vi "Add Injector Commands Section.vi"(8 "error in (no error)":errorcluster, 9 "Default Current Offset":dbl, 10 "Default Volt Offset":dbl, 11 "Injector Section ptr":T1=18446744073709551615 format="%.0x") -> (0 "error out":errorcluster, 3 "Parent Ref out":T1 format="%.0x")   [LabVIEW 2019, in "Fuel Injector Analysis Addon System Explorer.lvlib"]
uses:
  Fuel Injector Analysis Addon System Explorer.lvlib
  <vilib>/NI VeriStand/Custom Device API/Custom Device Item Ref.ctl
  <vilib>/NI VeriStand/Custom Device API/Custom Device Channel.ctl
  <vilib>/NI VeriStand/Custom Device API/Custom Device Channel Type.ctl
  Addon Shared/SubVIs/Constants.vi
  <vilib>/NI VeriStand/Custom Device API/Custom Device API.lvlib
  Addon Shared/Fuel Injector Analysis Addon Shared.lvlib
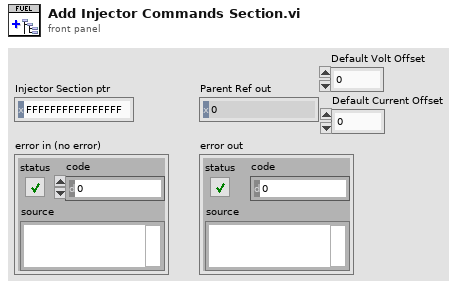
[diagram p1: front panel]
types:
  T1 = typedef "Custom Device API.lvlib/Custom Device Item Ref.ctl" = u64
  T2 = typedef "Custom Device API.lvlib/Custom Device Channel.ctl" = cluster{"Type":T3, "Units":string, "Default Value":dbl, "Faultable":bool, "Scalable":bool}
  T3 = typedef "Custom Device API.lvlib/Custom Device Channel Type.ctl" = enum16{"Input", "Output"}
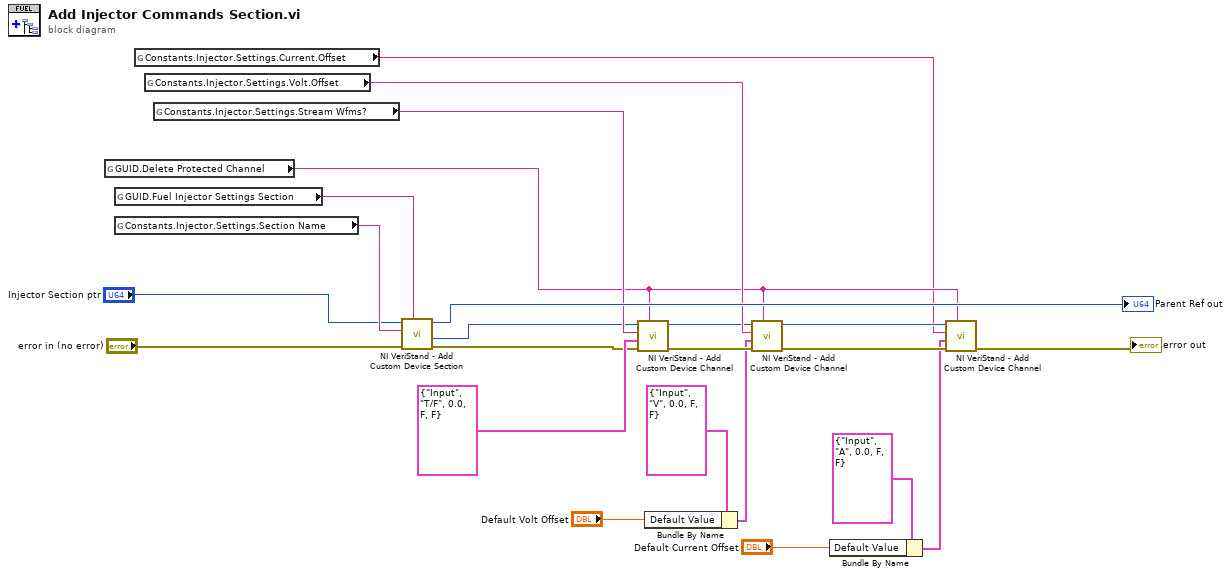
[diagram p0: block diagram]
diagram:
  n1 = global read "Constants.vi" "GUID.Delete Protected Channel"() -> (w8:string)
  n2 = global read "Constants.vi" "GUID.Fuel Injector Settings Section"() -> (w20:string)
  n3 = global read "Constants.vi" "Constants.Injector.Settings.Section Name"() -> (w19:string)
  n4 = global read "Constants.vi" "Constants.Injector.Settings.Current.Offset"() -> (w7:string)
  n5 = global read "Constants.vi" "Constants.Injector.Settings.Volt.Offset"() -> (w15:string)
  n6 = global read "Constants.vi" "Constants.Injector.Settings.Stream Wfms?"() -> (w21:string)
  n7 = call <vilib>:"NI VeriStand - Add Custom Device Section.vi"("GUID (Default Section)"=w20, "error in (no error)"="error in (no error)", "Section Name"=w19, "Parent Ref in"="Injector Section ptr") -> ("error out"=w13:errorcluster, "Section Ptr"=w12:T1, "Parent Ref out"=→"Parent Ref out":T1)  [unwired: 4 in, 1 out]
  n8 = call <vilib>:"NI VeriStand - Add Custom Device Channel.vi"("GUID (Default Channel)"=w8, "error in (no error)"=w13, "Channel"=T2 {"Type"=enum."Input", "Units"="T/F", "Default Value"=0.0, "Faultable"=FALSE, "Scalable"=FALSE}, "Channel Name"=w21, "Parent Ref in"=w12) -> ("error out"=w16:errorcluster, "Parent Ref out"=w14:T1)  [unwired: 3 in, 2 out]
  n9 = Bundle By Name(cluster=T2 {"Type"=enum."Input", "Units"="V", "Default Value"=0.0, "Faultable"=FALSE, "Scalable"=FALSE} ("Channel"), "Default Value"="Default Volt Offset") -> (w5:T2)
  n10 = call <vilib>:"NI VeriStand - Add Custom Device Channel.vi"("GUID (Default Channel)"=w8, "error in (no error)"=w16, "Channel"=w5, "Channel Name"=w15, "Parent Ref in"=w14) -> ("error out"=w11:errorcluster, "Parent Ref out"=w9:T1)  [unwired: 3 in, 2 out]
  n11 = Bundle By Name(cluster=T2 {"Type"=enum."Input", "Units"="A", "Default Value"=0.0, "Faultable"=FALSE, "Scalable"=FALSE} ("Channel"), "Default Value"="Default Current Offset") -> (w3:T2)
  n12 = call <vilib>:"NI VeriStand - Add Custom Device Channel.vi"("GUID (Default Channel)"=w8, "error in (no error)"=w11, "Channel"=w3, "Channel Name"=w7, "Parent Ref in"=w9) -> ("error out"=→"error out":errorcluster)  [unwired: 3 in, 3 out]
